vi "Status.vi"(7 "Reference":refnum<vi>, 10 "error in (no error)":errorcluster, 11 "Status":string) -> (2 "error out":errorcluster)   [LabVIEW 2019, in "Build.lvlib"]
uses:
  Build.lvlib
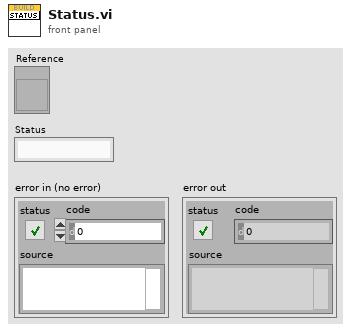
[diagram p1: front panel]
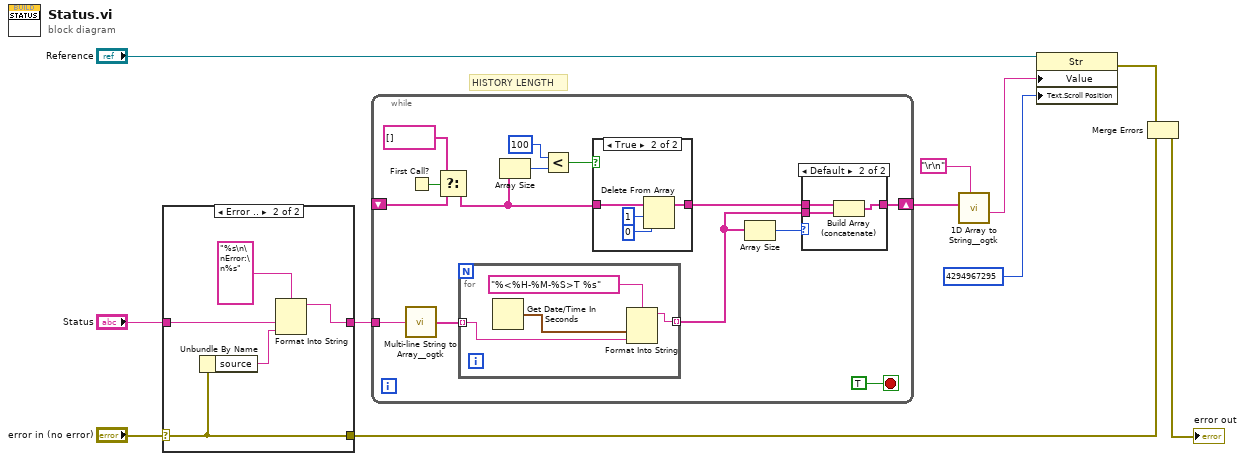
[diagram p0: block diagram]
diagram:
  # "HISTORY LENGTH"
  n1 = case shown="Error .." "error in (no error)" {
    selector: "error in (no error)" -> [w12 w14]
    tunnel: "Status" -> [w13 w15]
    tunnel: [w13 w17] -> w7
    tunnel: [w12 w14] -> w4
    frame No Error {
    }
    frame Error {
      n2 = Unbundle By Name(w14) -> ("source"=w16:string)
      n3 = Format Into String(format string="%s\n\nError:\n%s", w15, w16) -> (resulting string=w17:string)  [unwired: 2 in, 1 out]
    }
  }
  n4 = while {
    tunnel: w7 -> [w22]
    shift-right: [w29] -> w3
    shift-left: _ -> [w25]
    stop <- TRUE stop-if-true
    n5 = call <userlib>:"Multi-line String to Array__ogtk.vi"("string"=w22) -> ("lines"=w21:string[])
    n6 = First Call?() -> (First Call?: T/F=w26:bool)
    n7 = Select(t=string[] [], s=w26, f=w25) -> (s? t:f=w24:string[])
    n8 = for {
      tunnel: [w35] -> w20 mode=indexing
      tunnel: w21 -> [w34] mode=indexing
      n9 = Get Date/Time In Seconds() -> (seconds since 1Jan1904=w33:timestamp)
      n10 = Format Into String(format string="%<%H-%M-%S>T %s", w33, w34) -> (resulting string=w35:string)  [unwired: 2 in, 1 out]
    }
    n11 = Array Size(array=w24) -> (size(s)=w31:i32)
    n12 = Less?(x=100 ("length"), y=w31) -> (x < y?=w28:bool)
    n13 = case shown="True" w28 {
      tunnel: w24 -> [w37 w38]
      tunnel: [w37 w40] -> w32
      frame False {
      }
      frame True {
        n14 = Delete From Array(array=w38, length=1, index=0) -> (array with subset deleted=w40:string[])  [unwired: 1 out]
      }
    }
    n15 = Array Size(array=w20) -> (size(s)=w19:i32)
    n16 = case shown="Default" w19 {
      tunnel: w32 -> [w42 w43]
      tunnel: [w42 w45] -> w29
      tunnel: w20 -> [_ w44]
      frame 0 {
      }
      frame Default {
        n17 = Build Array (concatenate)(w43, w44) -> (w45:string[])
      }
    }
  }
  n18 = call <userlib>:"1D Array to String__ogtk.vi"("delimiter (Tab)"="\r\n", "Array of Strings"=w3) -> ("delimited string"=w1:string)  [unwired: 9 in]
  n19 = property class="Str"(reference="Reference", "Value"=w1, "Text.Scroll Position"=u32 4294967295) -> (error out=w6:errorcluster)  [unwired: 1 in, 1 out]
  n20 = Merge Errors(w6, w4) -> (→"error out":errorcluster)
